vi "conVert.vi"(0 "InstrumentID":u32, 2 "V scale":T1 {"Coupling" items=["DC 1 MOhm", "AC 1 MOhm", "DC 50 Ohm", "AC 50 OHM"]; "Offset" format="%.2f"}, 3 "error in":errorcluster, 4 "Channel (1)":i32=1) -> (5 "Status":i32 format="%.0x", 7 "error out":errorcluster)   [LabVIEW 2022 SP3]
uses:
  <instrlib>/Acqiris Dx/Acqiris Dx.lvlib
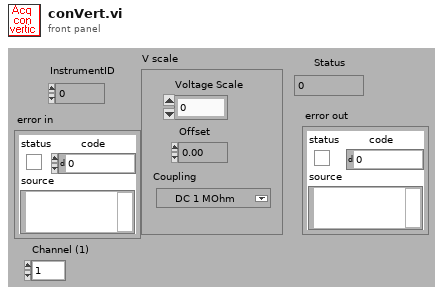
[diagram p1: front panel]
types:
  T1 = cluster{"Voltage Scale":dbl, "Offset":dbl, "Coupling":u16}
  T2 = enum32{"no bandwidth limit", "BWL 25 MHz", "BWL 700 MHz", "BWL 200 MHz", "BWL 20 MHz", "BWL 35 MHz"}
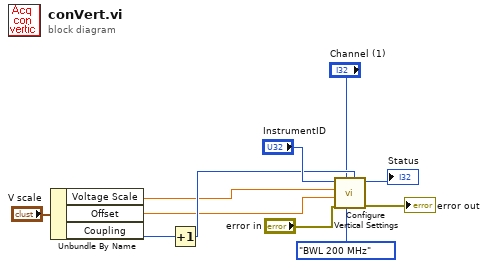
[diagram p0: block diagram]
diagram:
  n1 = Unbundle By Name("V scale") -> ("Voltage Scale"=w2:dbl, "Offset"=w1:dbl, "Coupling"=w8:u16)
  n2 = Increment(x=w8) -> (x+1=w7:u16)
  n3 = call <instrlib>:"Configure Vertical Settings.vi"("Coupling (1: DC, 1 MOhm)"=w7, "Bandwidth (0: no limit)"=T2."BWL 200 MHz", "Channel (1)"="Channel (1)", "error in (no error)"="error in", "Offset (0 V)"=w1, "Full Scale (5.0 V)"=w2, "Instrument ID"="InstrumentID") -> ("error out"=→"error out":errorcluster, "dup Instrument ID"=→"Status":u32)  [unwired: 3 out]
